vi "Main.vi"() -> ()   [LabVIEW 2019]
uses:
  <vilib>/numeric/Random Number (Range) U64.vi
  <vilib>/numeric/sub_Random U32.vi
  <vilib>/Utility/file.llb/Write Delimited Spreadsheet (I64).vi
  <vilib>/Utility/file.llb/Read Delimited Spreadsheet (I64).vi
  <vilib>/vision/NI_Vision_Development_Module.lvlib
panel:
  out "Numeric":ext=1000000000.0
  out "Image 3":T1(plugin-control)
  out "Image 5":T1(plugin-control)
  out "Image 4":T1(plugin-control)
  out "Image 2":T1(plugin-control)
  out "Image":T1(plugin-control)
  in  "file path":path
  in  "File Path":path
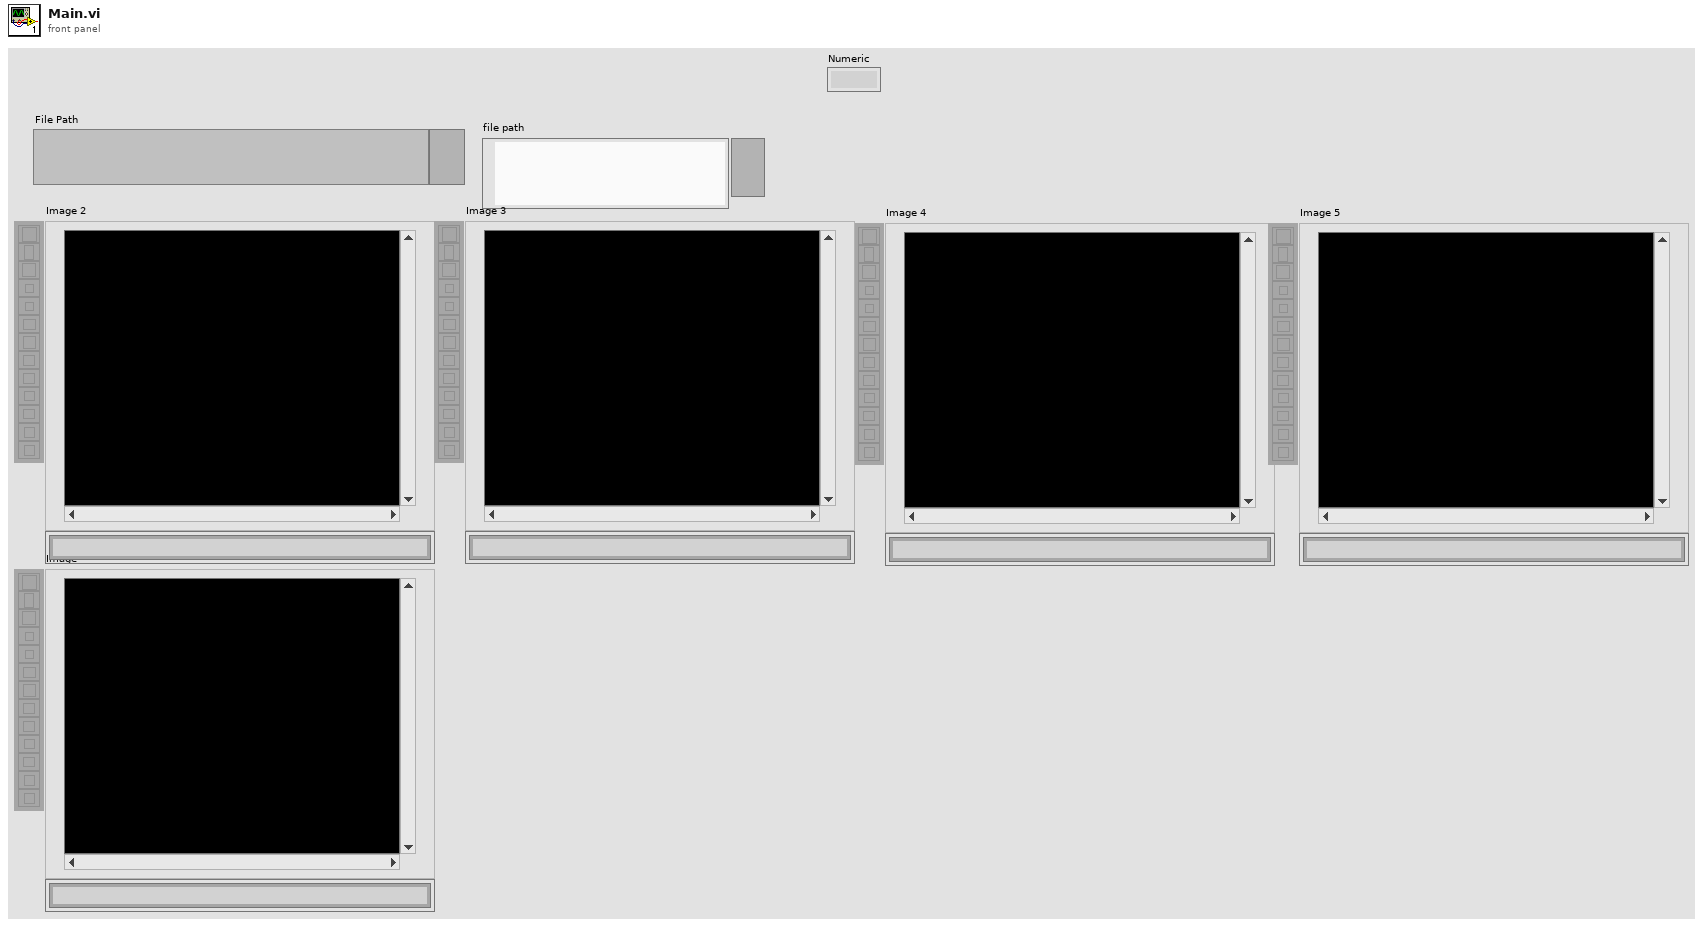
[diagram p1: front panel]
types:
  T1 = typedef "IMAQ Image.ctl" = refnum<image>
  T2 = typedef "Image Type" = u32
  T3 = cluster{"Image Dst Out":T1, cluster{"y":i32, "y":i32}}
  T4 = cluster{cluster{i32, i32}, cluster{i32, i32, i32}, i32}
  T5 = cluster{"New Image":T1, cluster{"y":i32, "y":i32}}
  T6 = cluster{cluster{"x":i32, "y":i32}, cluster{"r":i32, "g":i32, "b":i32}, "s":i32}
  T7 = cluster{"Numeric":i64, "Numeric":i64, "Numeric":i64}
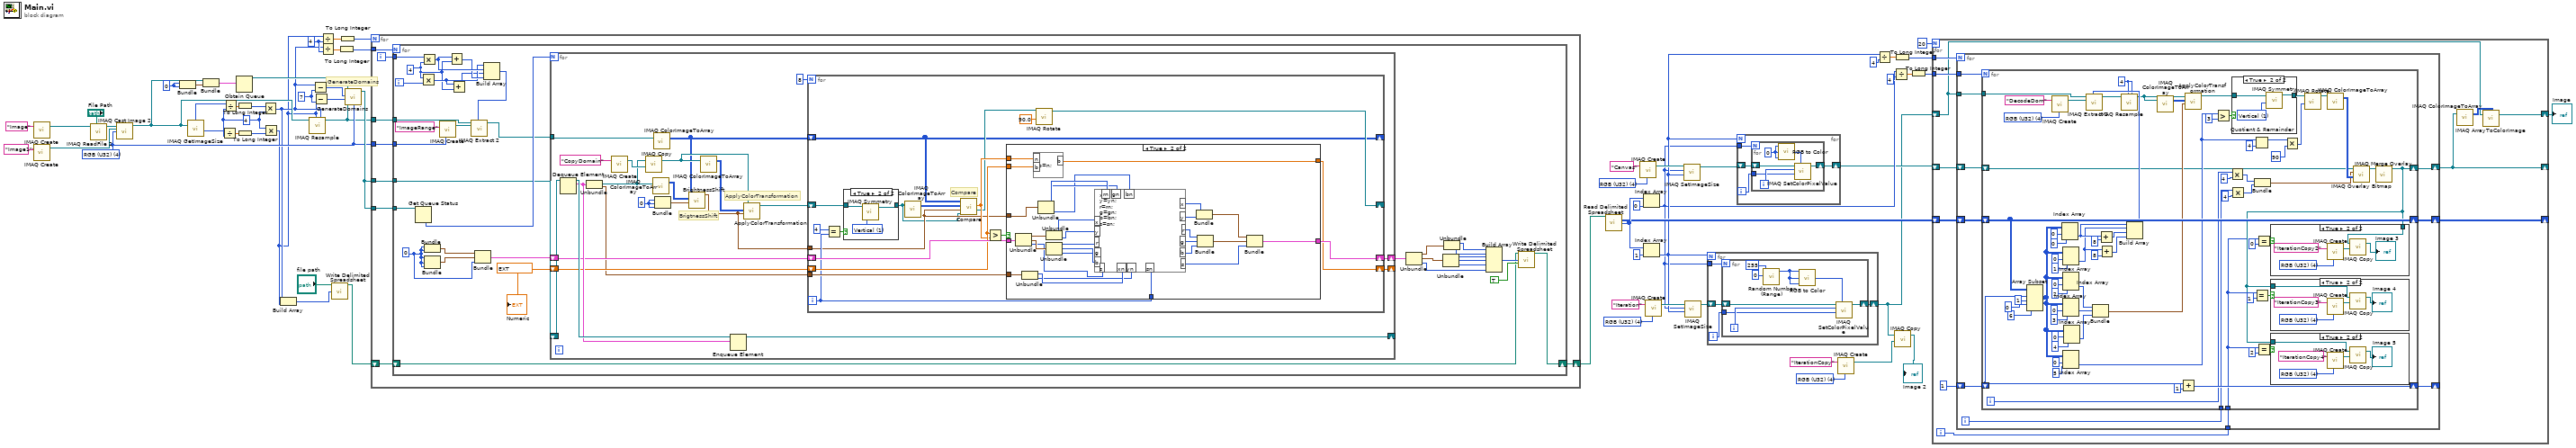
[diagram p0: block diagram]
diagram:
  w3 = T2 4 items=["Grayscale (U8)", "Grayscale (I16)", "Grayscale (SGL)", "Complex (CSG)", "RGB (U32)", "HSL (U32)", "RGB (U64)", "Grayscale (U16)"] ("Image Type")
  w24 = T2 4 items=["Grayscale (U8)", "Grayscale (I16)", "Grayscale (SGL)", "Complex (CSG)", "RGB (U32)", "HSL (U32)", "RGB (U64)", "Grayscale (U16)"] ("Image Type")
  w27 = T2 4 items=["Grayscale (U8)", "Grayscale (I16)", "Grayscale (SGL)", "Complex (CSG)", "RGB (U32)", "HSL (U32)", "RGB (U64)", "Grayscale (U16)"] ("Image Type")
  w38 = T2 4 items=["Grayscale (U8)", "Grayscale (I16)", "Grayscale (SGL)", "Complex (CSG)", "RGB (U32)", "HSL (U32)", "RGB (U64)", "Grayscale (U16)"] ("Image Type")
  w42 = 4 ("y")
  w48 = 7 ("y")
  w47 = 0 ("y")
  w58 = 4 ("y")
  # "GenerateDomains"
  n1 = call "IMAQ Create"("Image Name"="Image1") -> ("New Image"=w19:T1)  [unwired: 4 in, 1 out]
  n2 = call "IMAQ Create"("Image Name"="Image") -> ("New Image"=w40:T1)  [unwired: 4 in, 1 out]
  n3 = call "IMAQ ReadFile 2"("File Path"="File Path", "Image"=w40) -> ()  [unwired: 5 in, 5 out]
  n4 = call "IMAQ Cast Image 2"("Image Src"=w40, "Image Dst"=w19, "Image Type"=w38) -> ("Image Dst Out"=w39:T1)  [unwired: 11 in, 1 out]
  n5 = Bundle("y"=w47, "y"=w47) -> (w55:cluster{"y":i32, "y":i32})  [unwired: 1 in]
  n6 = call "IMAQ GetImageSize"("Image"=w39) -> ("Y Resolution"=w52:i32, "X Resolution"=w51:i32)  [unwired: 3 in, 1 out]
  n7 = Bundle("Image Dst Out"=w39, w55) -> (w54:T3)  [unwired: 1 in]
  n8 = Divide(x=w52, y=w58) -> (x/y=w60:dbl)
  n9 = Divide(x=w51, y=w58) -> (x/y=w59:dbl)
  n10 = Obtain Queue(element data type=w54) -> (queue out=w49:refnum<queue>)  [unwired: 4 in, 2 out]
  n11 = To Long Integer(number=w59) -> (32bit integer=w56:i32)
  n12 = To Long Integer(number=w60) -> (32bit integer=w57:i32)
  n13 = Multiply(x=w56, y=w58) -> (x*y=w36:i32)
  n14 = Multiply(x=w58, y=w57) -> (x*y=w35:i32)
  n15 = Build Array(w36, w35) -> (w34:i32[])
  n16 = call "IMAQ Resample"("X Resolution"=w36, "Y Resolution"=w35, "Image Src"=w39) -> ("Image Dst Out"=w22:T1)  [unwired: 7 in, 1 out]
  n17 = Subtract(x=w36, y=w48) -> (x-y=w50:i32)
  n18 = Subtract(x=w35, y=w48) -> (x-y=w53:i32)
  n19 = Divide(x=w35, y=w42) -> (x/y=w45:dbl)
  n20 = Divide(x=w36, y=w42) -> (x/y=w44:dbl)
  n21 = call-poly <vilib>:"Write Delimited Spreadsheet.vi"("file path (dialog if empty)"="file path", "1D data"=w34) -> ("new file path (Not A Path if cancelled)"=w33:path)  [unwired: 12 in, 1 out]
  n22 = To Long Integer(number=w44) -> (32bit integer=w43:i32)
  n23 = To Long Integer(number=w45) -> (32bit integer=w46:i32)
  n24 = call "GenerateDomains.vi"("Image Dst Out"=w22, "Image Type"=w38, "Numeric 2"=w53, "Numeric"=w50, "Queue in"=w49) -> ("Queue out"=w41:refnum<queue>)  [unwired: 6 in]
  n25 = for {
    N: w46 -> [_]
    tunnel: w43 -> [w70]
    tunnel: w22 -> [w68]
    tunnel: w41 -> [w67]
    tunnel: w38 -> [w66]
    tunnel: w41 -> [w65]
    shift-right: [w64] -> w32
    shift-left: w33 -> [w63]
    i -> [w69]
    n26 = for {
      N: w70 -> [_]
      tunnel: w69 -> [w103]
      tunnel: w68 -> [w94]
      tunnel: w67 -> [w92]
      tunnel: w66 -> [w93]
      tunnel: w65 -> [w87]
      shift-right: [w73] -> w64
      shift-left: w63 -> [w72]
      i -> [w102]
      w71 = ext 1000000000.0
      w88 = 0
      w98 = 4 ("y")
      n27 = Get Queue Status(queue=w92) -> (# elements in queue=w91:i32)  [unwired: 2 in, 7 out]
      n28 = Multiply(x=w98, y=w102) -> (x*y=w99:i32)
      n29 = Multiply(x=w103, y=w98) -> (x*y=w101:i32)
      n30 = Bundle(w88, w88) -> (w90:cluster{i32, i32})  [unwired: 1 in]
      n31 = Bundle(w88, w88, w88) -> (w89:cluster{i32, i32, i32})  [unwired: 1 in]
      n32 = call "IMAQ Create"("Image Name"="ImageRange", "Image Type"=w93) -> ("New Image"=w95:T1)  [unwired: 3 in, 1 out]
      n33 = Add(x=w101, y=w98) -> (x+y=w100:i32)
      n34 = Add(x=w99, y=w98) -> (x+y=w97:i32)
      n35 = Bundle(w90, w89, w88) -> (w85:T4)  [unwired: 1 in]
      n36 = Build Array(w99, w101, w97, w100) -> (w96:i32[])
      n37 = call "IMAQ Extract 2"("Optional Rectangle"=w96, "Image Dst"=w95, "Image Src"=w94) -> ("Image Dst Out"=w86:T1)  [unwired: 7 in, 1 out]
      n38 = for {
        N: w91 -> [_]
        tunnel: w86 -> [w126]
        shift-right: [w114] -> _
        shift-left: w87 -> [w115]
        shift-right: [w108] -> w84
        shift-left: w85 -> [w109]
        shift-right: [w106] -> _
        shift-left: w71 -> [w107]
        w125 = 0
        # "ApplyColorTransformation"
        # "BrigtnessShift"
        n39 = Dequeue Element(queue=w115) -> (queue out=w117:refnum<queue>, element=w116:T5)  [unwired: 2 in, 2 out]
        n40 = Unbundle(w116) -> ("New Image"=w118:T1, w105:cluster{"y":i32, "y":i32})
        n41 = call "IMAQ Create"("Image Name"="CopyDomain") -> ("New Image"=w121:T1)  [unwired: 4 in, 1 out]
        n42 = call "IMAQ Copy"("Image Dst"=w121, "Image Src"=w118) -> ("Image Dst Out"=w119:T1)  [unwired: 4 in, 1 out]
        n43 = call "IMAQ ColorImageToArray"("Image"=w118) -> ("Image Pixels (U32)"=w123:u32[][])  [unwired: 3 in, 2 out]
        n44 = call "IMAQ ColorImageToArray"("Image"=w126) -> ("Image Pixels (U32)"=w111:u32[][])  [unwired: 3 in, 2 out]
        n45 = Bundle(w125, w125, w125) -> (w124:cluster{i32, i32, i32})  [unwired: 1 in]
        n46 = call "BrightnessShift.vi"("Cluster in"=w124, "Image Pixels (U32)"=w123, "Image Pixels (U32) 2"=w111) -> ("Cluster out"=w110:cluster{i32, i32, i32})  [unwired: 8 in]
        n47 = call "IMAQ ColorImageToArray"("Image"=w119) -> ("Image Pixels (U32)"=w120:u32[][])  [unwired: 3 in, 2 out]
        n48 = Enqueue Element(queue=w117, element=w116) -> (queue out=w114:refnum<queue>)  [unwired: 2 in, 2 out]
        n49 = call "ApplyColorTransformation.vi"("Cluster in"=w110, "Image Pixels (U32)"=w120, "Refnum in"=w119) -> ("Refnum out"=w112:T1)  [unwired: 8 in]
        n50 = for {
          N: 8 -> [_]
          shift-right: [w141] -> _
          shift-left: w112 -> [w140]
          shift-right: [w127] -> _
          shift-left: w111 -> [w127]
          tunnel: w110 -> [w132]
          shift-right: [w137] -> w108
          shift-left: w109 -> [w138]
          shift-right: [w131] -> w106
          shift-left: w107 -> [w136]
          tunnel: w105 -> [w134]
          i -> [w133]
          # "Compare"
          n51 = Equal?(x=4, y=w133) -> (x = y?=w143:bool)
          n52 = case shown="True" w143 {
            tunnel: w140 -> [w176 w179]
            tunnel: [w176 w177] -> w130
            frame False {
            }
            frame True {
              w178 = u32 1 items=["Horizontal", "Vertical", "Central", "1st Diagonal", "2nd Diagonal"] ("Type of Symmetry")
              n53 = call "IMAQ Symmetry"("Type of Symmetry"=w178, "Image Src"=w179) -> ("Image Dst Out"=w177:T1)  [unwired: 3 in, 1 out]
            }
          }
          n54 = call "IMAQ ColorImageToArray"("Image"=w130) -> ("Image Pixels (U32)"=w142:u32[][])  [unwired: 3 in, 2 out]
          n55 = call "Compare.vi"("Image"=w130, "Cluster in"=w132, "Image Pixels (U32) in"=w142, "Image Pixels (U32) 3"=w127) -> ("Image Out"=w129:T1, "Numeric"=w135:ext)  [unwired: 6 in]
          n56 = Greater?(x=w136, y=w135) -> (0:w139:bool)
          n57 = case shown="True" w139 {
            tunnel: w138 -> [w146 w172]
            tunnel: [w146 w147] -> w137
            tunnel: w136 -> [w145 w175]
            tunnel: w135 -> [_ w174]
            tunnel: [w145 w173] -> w131
            tunnel: w134 -> [_ w161]
            tunnel: w133 -> [_ w157]
            tunnel: w132 -> [_ w165]
            frame False {
            }
            frame True {
              n58 = Unbundle(w172) -> (w171:cluster{i32, i32}, w170:cluster{i32, i32, i32}, w158:i32)
              n59 = Unbundle(w161) -> ("y"=w160:i32, "y"=w159:i32)
              n60 = formula code="b=n;"("b"=w175, "n"=w174) -> ("b"=w173:ext)
              n61 = Unbundle(w165) -> (w164:i32, w163:i32, w162:i32)
              n62 = Unbundle(w171) -> (w166:i32, w156:i32)
              n63 = Unbundle(w170) -> (w167:i32, w168:i32, w169:i32)
              n64 = formula code="x=xn;\ny=yn;\nr=rn;\ng=gn;\nb=bn;\ns=sn;"("y"=w156, "x"=w166, "r"=w167, "g"=w168, "b"=w169, "s"=w158, "rn"=w164, "gn"=w163, "bn"=w162, "xn"=w160, "yn"=w159, "sn"=w157) -> ("x"=w155:i32, "y"=w154:i32, "r"=w153:i32, "g"=w152:i32, "b"=w151:i32, "s"=w150:i32)
              n65 = Bundle("x"=w155, "y"=w154) -> (w148:cluster{"x":i32, "y":i32})  [unwired: 1 in]
              n66 = Bundle("r"=w153, "g"=w152, "b"=w151) -> (w149:cluster{"r":i32, "g":i32, "b":i32})  [unwired: 1 in]
              n67 = Bundle(w148, w149, "s"=w150) -> (w147:T6)  [unwired: 1 in]
            }
          }
          n68 = call "IMAQ Rotate"("Angle (degrees)"=sgl 90.0, "Image Src"=w129) -> ("Image Dst Out"=w141:T1)  [unwired: 8 in, 1 out]
        }
      }
      n69 = Unbundle(w84) -> (w83:cluster{i32, i32}, w82:cluster{i32, i32, i32}, w76:i32)
      n70 = Unbundle(w82) -> (w79:i32, w78:i32, w77:i32)
      n71 = Unbundle(w83) -> (w81:i32, w80:i32)
      n72 = Build Array(w81, w80, w79, w78, w77, w76) -> (w75:i32[])
      n73 = call-poly <vilib>:"Write Delimited Spreadsheet.vi"("file path (dialog if empty)"=w72, "1D data"=w75, "append to file? (new file:F)"=TRUE) -> ("new file path (Not A Path if cancelled)"=w73:path)  [unwired: 11 in, 1 out]
      "Numeric" <- w71
    }
  }
  n74 = call-poly <vilib>:"Read Delimited Spreadsheet.vi"("file path (dialog if empty)"=w32) -> ("all rows"=w11:i64[][], "first row"=w29:i64[])  [unwired: 9 in, 4 out]
  n75 = call "IMAQ Create"("Image Name"="Canvas", "Image Type"=w27) -> ("New Image"=w26:T1)  [unwired: 3 in, 1 out]
  n76 = Index Array(array=w29, index=0) -> (element=w8:i64)
  n77 = Index Array(array=w29, index=1) -> (element=w9:i64)
  n78 = call "IMAQ Create"("Image Name"="Iteration", "Image Type"=w24) -> ("New Image"=w23:T1)  [unwired: 3 in, 1 out]
  n79 = call "IMAQ SetImageSize"("Y Resolution"=w9, "X Resolution"=w8, "Image"=w26) -> ("Image Out"=w7:T1)  [unwired: 2 in, 1 out]
  n80 = call "IMAQ SetImageSize"("Y Resolution"=w9, "X Resolution"=w8, "Image"=w23) -> ("Image Out"=w21:T1)  [unwired: 2 in, 1 out]
  n81 = for {
    N: w9 -> [_]
    shift-right: [w182] -> w5
    shift-left: w21 -> [w183]
    tunnel: w8 -> [w180]
    i -> [w181]
    n82 = for {
      N: w180 -> [_]
      shift-right: [w186] -> w182
      shift-left: w183 -> [w189]
      tunnel: w181 -> [w187]
      i -> [w188]
      n83 = call-poly <vilib>:"Random Number (Range).vi"("lower bound (0)"=u64 0, "upper bound (100)"=u64 255) -> ("number"=w185:u64)  [unwired: 9 in]
      n84 = call <vilib>:"RGB to Color.vi"("B"=w185, "G"=w185, "R"=w185) -> ("Color"=w184:u32)
      n85 = call "IMAQ SetColorPixelValue"("Pixel Value (U32)"=w184, "Y Coordinate"=w187, "X Coordinate"=w188, "Image"=w189) -> ("Image Out"=w186:T1)  [unwired: 6 in, 1 out]
    }
  }
  n86 = for {
    N: w9 -> [_]
    shift-right: [w194] -> w6
    shift-left: w7 -> [w195]
    tunnel: w8 -> [w192]
    i -> [w193]
    n87 = for {
      N: w192 -> [_]
      shift-right: [w199] -> w194
      shift-left: w195 -> [w201]
      tunnel: w193 -> [w198]
      i -> [w200]
      w197 = u8 0 ("R")
      n88 = call <vilib>:"RGB to Color.vi"("B"=w197, "G"=w197, "R"=w197) -> ("Color"=w196:u32)
      n89 = call "IMAQ SetColorPixelValue"("Pixel Value (U32)"=w196, "Y Coordinate"=w198, "X Coordinate"=w200, "Image"=w201) -> ("Image Out"=w199:T1)  [unwired: 6 in, 1 out]
    }
  }
  n90 = call "IMAQ Create"("Image Name"="IterationCopy", "Image Type"=w3) -> ("New Image"=w2:T1)  [unwired: 3 in, 1 out]
  n91 = Divide(x=w9, y=i64 4) -> (x/y=w13:dbl)
  n92 = Divide(x=w8, y=i64 4) -> (x/y=w16:dbl)
  n93 = To Long Integer(number=w13) -> (32bit integer=w12:i32)
  n94 = call "IMAQ Copy"("Image Dst"=w2, "Image Src"=w5) -> ("Image Dst Out"=→"Image 2":T1)  [unwired: 4 in, 1 out]
  n95 = To Long Integer(number=w16) -> (32bit integer=w15:i32)
  n96 = for {
    N: 20 -> [_]
    tunnel: w15 -> [w211]
    tunnel: w12 -> [w210]
    shift-right: [w208] -> _
    shift-left: w11 -> [w209]
    shift-right: [w204] -> w10
    shift-left: w5 -> [w203]
    shift-right: [w205] -> _
    shift-left: w6 -> [w207]
    i -> [w202]
    n97 = for {
      N: w210 -> [_]
      shift-right: [w221] -> _
      shift-left: 1 -> [w222]
      tunnel: w211 -> [w220]
      shift-right: [w218] -> w208
      shift-left: w209 -> [w219]
      shift-right: [w215] -> w205
      shift-left: w207 -> [w216]
      tunnel: w203 -> [w214]
      tunnel: w202 -> [w213]
      i -> [w217]
      n98 = for {
        N: w220 -> [_]
        shift-right: [w289] -> w221
        shift-left: w222 -> [w284]
        shift-right: [w280] -> w218
        shift-left: w219 -> [w280]
        tunnel: w217 -> [w240]
        shift-right: [w224] -> w215
        shift-left: w216 -> [w235]
        tunnel: w214 -> [w233]
        tunnel: w213 -> [w223]
        i -> [w242]
        w259 = 4 ("X Resolution")
        w286 = T2 4 items=["Grayscale (U8)", "Grayscale (I16)", "Grayscale (SGL)", "Complex (CSG)", "RGB (U32)", "HSL (U32)", "RGB (U64)", "Grayscale (U16)"] ("Image Type")
        n99 = Array Subset(array=w280, index (row)=w284, length (row)=1 ("length"), index (col)=0 ("index"), length (col)=6 ("length")) -> (w271:i64[][])
        n100 = call "IMAQ Create"("Image Name"="DecodeDom", "Image Type"=w286) -> ("New Image"=w285:T1)  [unwired: 3 in, 1 out]
        n101 = Index Array(array=w271, index (row)=0, index (col)=0 ("disabled index (col)")) -> (element=w266:i64)
        n102 = Index Array(array=w271, index (row)=0, index (col)=3 ("disabled index (col)")) -> (element=w257:i64)
        n103 = Index Array(array=w271, index (row)=0, index (col)=1 ("disabled index (col)")) -> (element=w263:i64)
        n104 = Index Array(array=w271, index (row)=0, index (col)=2 ("disabled index (col)")) -> (element=w258:i64)
        n105 = Index Array(array=w271, index (row)=0, index (col)=5 ("disabled index (col)")) -> (element=w249:i64)
        n106 = Index Array(array=w271, index (row)=0, index (col)=4 ("disabled index (col)")) -> (element=w256:i64)
        n107 = Bundle("Numeric"=w258, "Numeric"=w257, "Numeric"=w256) -> (w253:T7)  [unwired: 1 in]
        n108 = Add(x=w266, y=i64 8) -> (x+y=w264:i64)
        n109 = Add(x=w263, y=i64 8) -> (x+y=w261:i64)
        n110 = Build Array(w266, w263, w264, w261) -> (w260:i64[])
        n111 = call "IMAQ Extract 2"("Optional Rectangle"=w260, "Image Dst"=w285, "Image Src"=w233) -> ("Image Dst Out"=w231:T1)  [unwired: 7 in, 1 out]
        n112 = call "IMAQ Resample"("X Resolution"=w259, "Y Resolution"=w259, "Image Src"=w231) -> ("Image Dst Out"=w255:T1)  [unwired: 7 in, 1 out]
        n113 = call "IMAQ ColorImageToArray"("Image"=w255) -> ("Image Pixels (U32)"=w254:u32[][])  [unwired: 3 in, 2 out]
        n114 = Add(x=w284, y=1) -> (x+y=w289:i32)
        n115 = call "ApplyColorTransformation.vi"("Cluster in"=w253, "Image Pixels (U32)"=w254, "Refnum in"=w255) -> ("Refnum out"=w250:T1)  [unwired: 8 in]
        n116 = Greater?(x=w249, y=i64 3) -> (0:w251:bool)
        n117 = Multiply(x=w242, y=4) -> (x*y=w238:i32)
        n118 = Multiply(x=w240, y=4) -> (x*y=w237:i32)
        n119 = case shown="True" w251 {
          tunnel: w250 -> [w305 w308]
          tunnel: [w305 w306] -> w244
          frame False {
          }
          frame True {
            w307 = u32 1 items=["Horizontal", "Vertical", "Central", "1st Diagonal", "2nd Diagonal"] ("Type of Symmetry")
            n120 = call "IMAQ Symmetry"("Type of Symmetry"=w307, "Image Src"=w308) -> ("Image Dst Out"=w306:T1)  [unwired: 3 in, 1 out]
          }
        }
        n121 = Quotient & Remainder(x=w249, y=i64 4) -> (x-y*floor(x/y)=w246:i64)  [unwired: 1 out]
        n122 = Equal?(x=w223, y=1) -> (x = y?=w228:bool)
        n123 = Bundle(w238, w237) -> (w236:cluster{i32, i32})  [unwired: 1 in]
        n124 = Equal?(x=w223, y=0) -> (x = y?=w230:bool)
        n125 = Equal?(x=w223, y=2) -> (x = y?=w226:bool)
        n126 = Multiply(x=w246, y=90) -> (x*y=w245:i64)
        n127 = call "IMAQ Rotate"("Angle (degrees)"=w245, "Image Src"=w244) -> ("Image Dst Out"=w234:T1)  [unwired: 8 in, 1 out]
        n128 = call "IMAQ ColorImageToArray"("Image"=w234) -> ("Image Pixels (U32)"=w243:u32[][])  [unwired: 3 in, 2 out]
        n129 = call "IMAQ Overlay Bitmap"("Bitmap"=w243, "Top Left Point"=w236, "Image"=w235) -> ("Image Out"=w232:T1)  [unwired: 7 in, 1 out]
        n130 = call "IMAQ Merge Overlay"("Image Src"=w232) -> ("Image Dst Out"=w224:T1)  [unwired: 9 in, 1 out]
        n131 = case shown="True" w230 {
          tunnel: w224 -> [_ w301]
          frame False {
          }
          frame True {
            w303 = T2 4 items=["Grayscale (U8)", "Grayscale (I16)", "Grayscale (SGL)", "Complex (CSG)", "RGB (U32)", "HSL (U32)", "RGB (U64)", "Grayscale (U16)"] ("Image Type")
            n132 = call "IMAQ Create"("Image Name"="IterationCopy2", "Image Type"=w303) -> ("New Image"=w302:T1)  [unwired: 3 in, 1 out]
            n133 = call "IMAQ Copy"("Image Dst"=w302, "Image Src"=w301) -> ("Image Dst Out"=→"Image 3":T1)  [unwired: 4 in, 1 out]
          }
        }
        n134 = case shown="True" w228 {
          tunnel: w224 -> [_ w295]
          frame False {
          }
          frame True {
            w298 = T2 4 items=["Grayscale (U8)", "Grayscale (I16)", "Grayscale (SGL)", "Complex (CSG)", "RGB (U32)", "HSL (U32)", "RGB (U64)", "Grayscale (U16)"] ("Image Type")
            n135 = call "IMAQ Create"("Image Name"="IterationCopy3", "Image Type"=w298) -> ("New Image"=w297:T1)  [unwired: 3 in, 1 out]
            n136 = call "IMAQ Copy"("Image Dst"=w297, "Image Src"=w295) -> ("Image Dst Out"=→"Image 4":T1)  [unwired: 4 in, 1 out]
          }
        }
        n137 = case shown="True" w226 {
          tunnel: w224 -> [_ w290]
          frame False {
          }
          frame True {
            w293 = T2 4 items=["Grayscale (U8)", "Grayscale (I16)", "Grayscale (SGL)", "Complex (CSG)", "RGB (U32)", "HSL (U32)", "RGB (U64)", "Grayscale (U16)"] ("Image Type")
            n138 = call "IMAQ Create"("Image Name"="IterationCopy4", "Image Type"=w293) -> ("New Image"=w292:T1)  [unwired: 3 in, 1 out]
            n139 = call "IMAQ Copy"("Image Dst"=w292, "Image Src"=w290) -> ("Image Dst Out"=→"Image 5":T1)  [unwired: 4 in, 1 out]
          }
        }
      }
    }
    n140 = call "IMAQ ColorImageToArray"("Image"=w205) -> ("Image Pixels (U32)"=w206:u32[][])  [unwired: 3 in, 2 out]
    n141 = call "IMAQ ArrayToColorImage"("Image Pixels (U32)"=w206, "Image"=w203) -> ("Image Out"=w204:T1)  [unwired: 3 in, 1 out]
  }
  "Image" <- w10
